vi "test9-LosslessRegisterStatusMultipleTimes.vi"(8 "error in (no error)":errorcluster, 11 "TestCase in":refnum<class "testcase-CSMStatusStateRegisterUnregister.lvclass">) -> (0 "error out":errorcluster, 3 "TestCase out":refnum<class "testcase-CSMStatusStateRegisterUnregister.lvclass">)   [LabVIEW 2017, in "testcase-CSMStatusStateRegisterUnregister.lvclass"]
uses:
  testcase-CSMStatusStateRegisterUnregister.lvclass
  src/user.lib/_NEVSTOP/Communicable State Machine(CSM)/_Support/Typedef/_CSM_List Module Scope.ctl
  bc269a46-fbd8-4fbd-ac76-06990d02385a.vi
  8d37a2f4-20d8-4102-818c-5a8acec6f80e.vi
  src/user.lib/_NEVSTOP/Communicable State Machine(CSM)/AdvanceAPI/CSM - Get Module Attribute.vi
  <vilib>/addons/_JKI Toolkits/VI Tester/TestCase.llb/TestCase.lvclass
  src/user.lib/_NEVSTOP/Communicable State Machine(CSM)/Communicable State Machine.lvlib
  C:/Program Files (x86)/National Instruments/LabVIEW 2017/vi.lib/addons/_JKI Toolkits/VI Tester/TestCase.llb/TestCase.lvclass
panel:
  out "error out 2":errorcluster
  out "LoopCount":i32
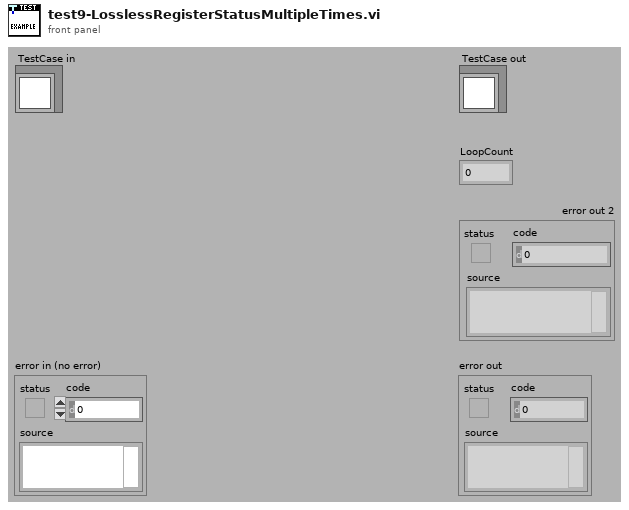
[diagram p1: front panel]
types:
  T1 = typedef "Communicable State Machine.lvlib/_CSM_List Module Scope.ctl" = enum16{"Normal", "System Only", "All"}
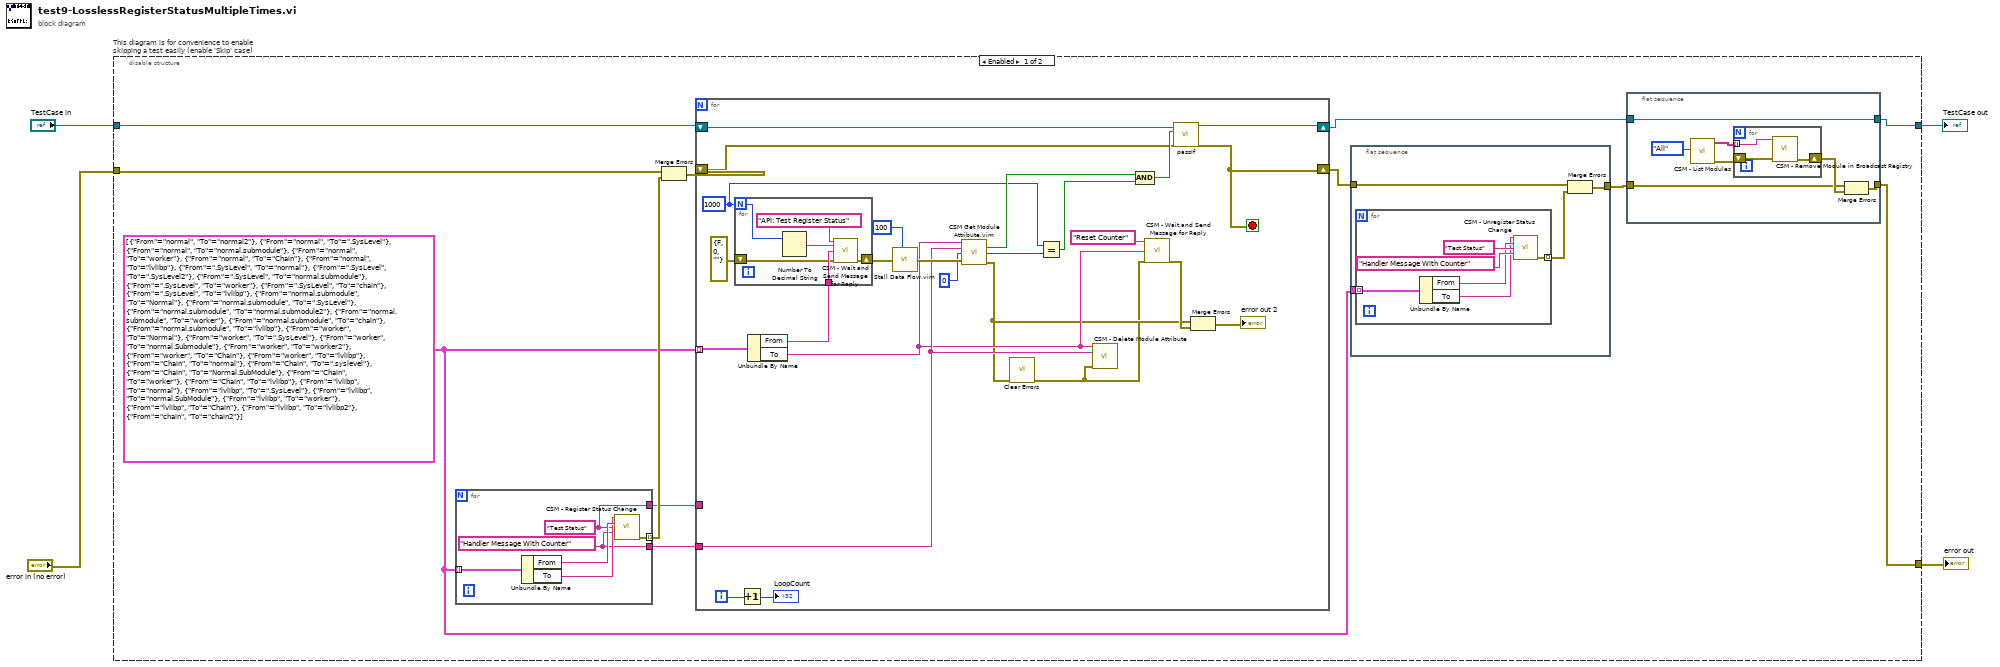
[diagram p0: block diagram]
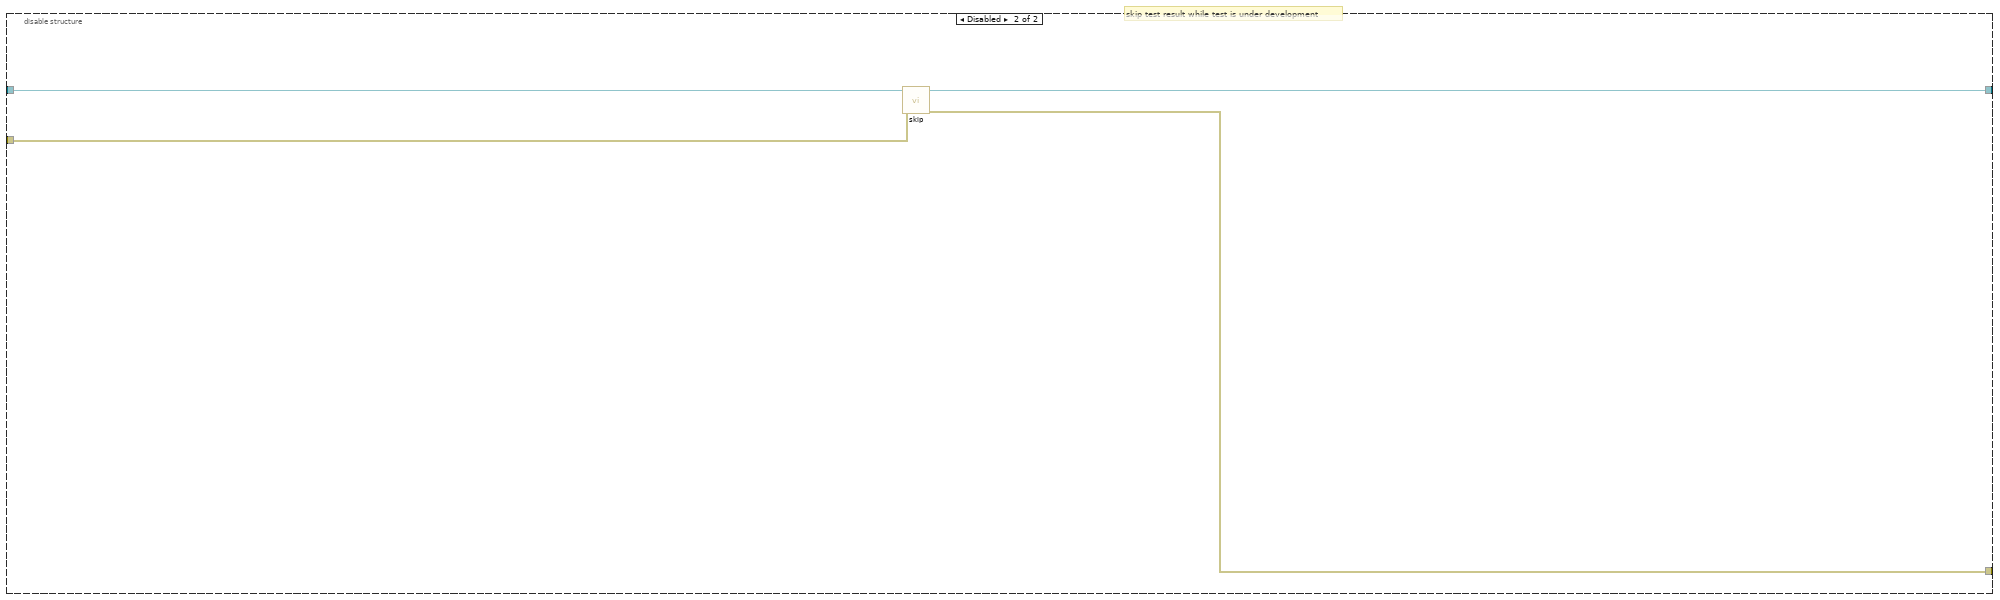
[diagram p2: hidden frame]
diagram:
  n1 = disable-structure "This diagram is for convenience to enable skipping a test easily (enable 'Skip' case)" shown="Enabled" {
    disable-tunnel: "TestCase in" -> [w16 w77]
    disable-tunnel: [w6 w75] -> w2
    disable-tunnel: [w9 w76] -> w1
    disable-tunnel: "error in (no error)" -> [w15 w74]
    frame Enabled {
      w12 = cluster{"From":string, "To":string}[] [{"From"="normal", "To"="normal2"}, {"From"="normal", "To"=".SysLevel"}, {"From"="normal", "To"="normal.submodule"}, {"From"="normal", "To"="worker"}, {"From"="normal", "To"="Chain"}, {"From"="normal", "To"="lvlibp"}, {"From"=".SysLevel", "To"="normal"}, {"From"=".SysLevel", "To"=".SysLevel2"}, {"From"=".SysLevel", "To"="normal.submodule"}, {"From"=".SysLevel", "To"="worker"}, {"From"=".SysLevel", "To"="chain"}, {"From"=".SysLevel", "To"="lvlibp"}, {"From"="normal.submodule", "To"="Normal"}, {"From"="normal.submodule", "To"=".SysLevel"}, {"From"="normal.submodule", "To"="normal.submodule2"}, {"From"="normal.submodule", "To"="worker"}, {"From"="normal.submodule", "To"="chain"}, {"From"="normal.submodule", "To"="lvlibp"}, {"From"="worker", "To"="Normal"}, {"From"="worker", "To"=".SysLevel"}, {"From"="worker", "To"="normal.Submodule"}, {"From"="worker", "To"="worker2"}, {"From"="worker", "To"="Chain"}, {"From"="worker", "To"="lvlibp"}, {"From"="Chain", "To"="normal"}, {"From"="Chain", "To"=".syslevel"}, {"From"="Chain", "To"="Normal.SubModule"}, {"From"="Chain", "To"="worker"}, {"From"="Chain", "To"="lvlibp"}, {"From"="lvlibp", "To"="normal"}, {"From"="lvlibp", "To"=".SysLevel"}, {"From"="lvlibp", "To"="normal.SubModule"}, {"From"="lvlibp", "To"="worker"}, {"From"="lvlibp", "To"="Chain"}, {"From"="lvlibp", "To"="lvlibp2"}, {"From"="chain", "To"="chain2"}]
      n2 = for {
        tunnel: w12 -> [w32] mode=indexing
        tunnel: [w29] -> w13 mode=indexing
        tunnel: [w28] -> w8
        tunnel: [w27] -> w5
        w27 = "Handler Message With Counter" ("Response Message (If \"\", Same as Source Message)")
        w28 = "Test Status" ("Status")
        n3 = Unbundle By Name(w32) -> ("From"=w31:string, "To"=w30:string)
        n4 = call "CSM - Register Status Change.vi"("CSM Name"=w30, "Source CSM Name (* as Default)"=w31, "Status"=w28, "Response Message (If \"\", Same as Source Message)"=w27) -> ("error out"=w29:errorcluster)  [unwired: 10 in, 1 out]
      }
      n5 = Merge Errors(w15, w13) -> (w14:errorcluster)
      n6 = for {
        tunnel: w12 -> [w67] mode=indexing
        shift-right: [w60] -> w7
        shift-left: w16 -> [w61]
        shift-right: [w57] -> w11
        shift-left: w14 -> [w58]
        tunnel: w8 -> [_]
        tunnel: w5 -> [w56]
        i -> [w55]
        stop <- w57 stop-if-true
        w50 = 1000
        n7 = Increment(x=w55) -> (x+1=→"LoopCount":i32)
        n8 = Unbundle By Name(w67) -> ("From"=w62:string, "To"=w47:string)
        n9 = for {
          N: w50 -> [w68]
          tunnel: w62 -> [w71]
          shift-right: [w72] -> w66
          shift-left: errorcluster {"status"=FALSE, "code"=0, "source"=""} ("error out") -> [w70]
          n10 = Number To Decimal String(number=w68) -> (decimal integer string=w69:string)  [unwired: 1 in]
          n11 = call "CSM - Wait and Send Message for Reply.vi"("State"="API: Test Register Status", "Arguments (\"\")"=w69, "Target Module"=w71, "Error In (No Error)"=w70) -> ("error out"=w72:errorcluster)  [unwired: 9 in, 2 out]
        }
        n12 = call "Stall Data Flow.vim"("value in"=w66, "milliseconds to wait"=u32 100) -> ("value out"=w64:errorcluster)  [unwired: 1 out]
        n13 = call "CSM Get Module Attribute.vim"("CSM Name"=w47, "Attribute"=w56, "Default Value (Empty Variant)"=u32 0, "Error In"=w64) -> ("Found"=w63:bool, "Value"=w51:u32, "error out"=w44:errorcluster)  [unwired: 7 in, 2 out]
        n14 = call <vilib>:"Clear Errors.vi"("error in (no error)"=w44) -> ("error out"=w43:errorcluster)  [unwired: 5 in, 1 out]
        n15 = Equal?(x=w50, y=w51) -> (x = y?=w49:bool)
        n16 = call "CSM - Delete Module Attribute.vi"("CSM Name"=w47, "Attribute"=w56, "Error In"=w43) -> ()  [unwired: 9 in, 4 out]
        n17 = Compound Arithmetic op=AND(w63, w49) -> (w59:bool)
        n18 = call "CSM - Wait and Send Message for Reply.vi"("State"="Reset Counter", "Target Module"=w47, "Error In (No Error)"=w43) -> ("error out"=w46:errorcluster)  [unwired: 10 in, 2 out]
        n19 = call-dynamic "passIf.vi"("error in (no error)"=w58, "pass"=w59, "TestCase in"=w61) -> ("error out"=w57:errorcluster, "TestCase out"=w60:refnum<class "testcase-CSMStatusStateRegisterUnregister.lvclass">)  [unwired: 7 in]
        n20 = Merge Errors(w44, w46) -> (→"error out 2":errorcluster)
      }
      n21 = flat-sequence {
        tunnel: w12 -> [w17]
        tunnel: w11 -> [w20]
        tunnel: [w19] -> w10
        frame #0 {
          n22 = for {
            tunnel: w17 -> [w21] mode=indexing
            tunnel: [w22] -> w18 mode=indexing
            n23 = Unbundle By Name(w21) -> ("From"=w24:string, "To"=w23:string)
            n24 = call "CSM - Unregister Status Change.vi"("CSM Name"=w23, "Source CSM Name (* as Default)"=w24, "Status"="Test Status", "Response Message (\"*\" as Default)"="Handler Message With Counter" ("Response Message (If \"\", Same as Source Message)")) -> ("error out"=w22:errorcluster)  [unwired: 10 in, 1 out]
          }
          n25 = Merge Errors(w20, w18) -> (w19:errorcluster)
        }
      }
      n26 = flat-sequence {
        tunnel: w10 -> [w35]
        tunnel: [w34] -> w9
        tunnel: [w33] -> w6
        tunnel: w7 -> [w33]
        frame #0 {
          n27 = call "CSM - List Modules.vi"("Scope (Normal)"=_CSM_List_Module_Scope."All") -> ("error out"=w37:errorcluster, "Module Names"=w38:string[])  [unwired: 9 in]
          n28 = for {
            tunnel: w38 -> [w42] mode=indexing
            shift-right: [w40] -> w39
            shift-left: w37 -> [w41]
            n29 = call "CSM - Remove Module in Broadcast Registry.vi"("CSM Name"=w42, "Error In"=w41) -> ("error out"=w40:errorcluster)  [unwired: 12 in, 1 out]
          }
          n30 = Merge Errors(w35, w39) -> (w34:errorcluster)
        }
      }
    }
    frame Disabled {
      # "skip test result while test is under development"
      n31 = call <vilib>:"skip.vi"("error in (no error)"=w74, "TestCase in"=w77) -> ("error out"=w76:errorcluster, "TestCase out"=w75:refnum<class "testcase-CSMStatusStateRegisterUnregister.lvclass">)  [unwired: 8 in]
    }
  }
  "error out" <- w1
  "TestCase out" <- w2
